vi "Run.vi"(8 "error in (no error)":errorcluster, 11 "Channel in":refnum<class "Channel.lvclass">) -> (0 "error out":errorcluster, 3 "Channel out":refnum<class "Channel.lvclass">)   [LabVIEW 2018, in "Channel.lvclass"]
doc: "Run the channel"
uses:
  Channel.lvclass
  Channel.lvclass/Channel.ctl
  Sim_Ixon_Ultra/Sim_Ixon_Ultra.lvclass
  C:/Users/Denis/Desktop/S4ACS/S4ACS/Simulated_CCD_Camera/Simulated Camera.lvclass
  State Machine/State Machine.lvclass
  Simulated_CCD_Camera/Simulated Camera.lvclass
  RxTx/RxTx.lvclass
  Server/Server.lvclass
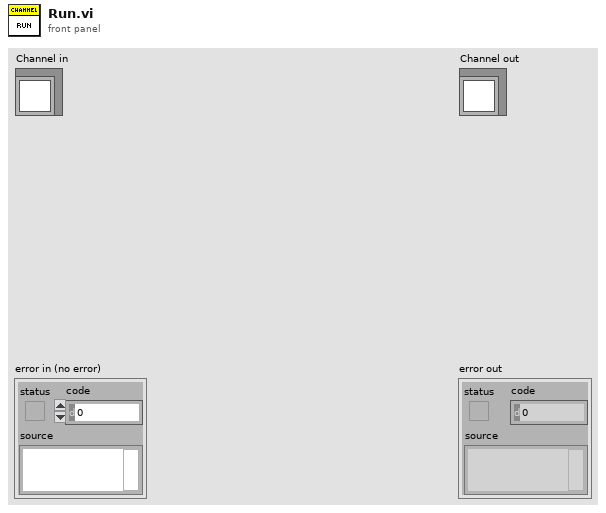
[diagram p1: front panel]
types:
  T1 = cluster{"PREAMP":u16, "READOUT_RATE":u16, "VERTICAL_SHIFT_SPEED":u16, "READ_MODE":u16, "VERTICAL_CLOCK_VOLTAGE":u16, "ACQUISITION_MODE":u16, "AD_CHANNEL":u16, "SHUTTER_TTL":u16, "SHUTTER_OPENING_TIME":u16, "SHUTTER_CLOSING_TIME":u16, "SHUTTER_MODE":u16, "TRIGGER_MODE":u16, "VBIN":u16, "INITIAL_LINE":u16, "INITIAL_COLUMN":u16, "FINAL_LINE":u16, "FINAL_COLUMN":u16, "HBIN":u16, "TEMP":u16, "COOLER_POWER_STATUS":u16}
  T2 = typedef "LVDateTimeRec.ctl" = cluster{"fractional second":dbl, "second":i32, "minute":i32, "hour":i32, "day of month":i32, "month":i32, "year":i32, "day of week":i32, "day of year":i32, "DST":i32}
  T3 = cluster{"Time Acq Started":u32, "Image delay":u64, "Last update - CCD config":timestamp, "SYSTEMTIME":T2, "Readout time":dbl, "Time acq finished":u32, "effective exptime":dbl}
  T4 = cluster{"FRAMES_DONE":u16, "CCD_STATUS":string, "CURRENT_TEMPERATURE":i16, "TEMPERATURE_STATUS":string, "FRAME_EXPOSURE_TIME":sgl, "SERIAL_NUMBER":u16, "ACQUIRING":bool, "POWER":bool}
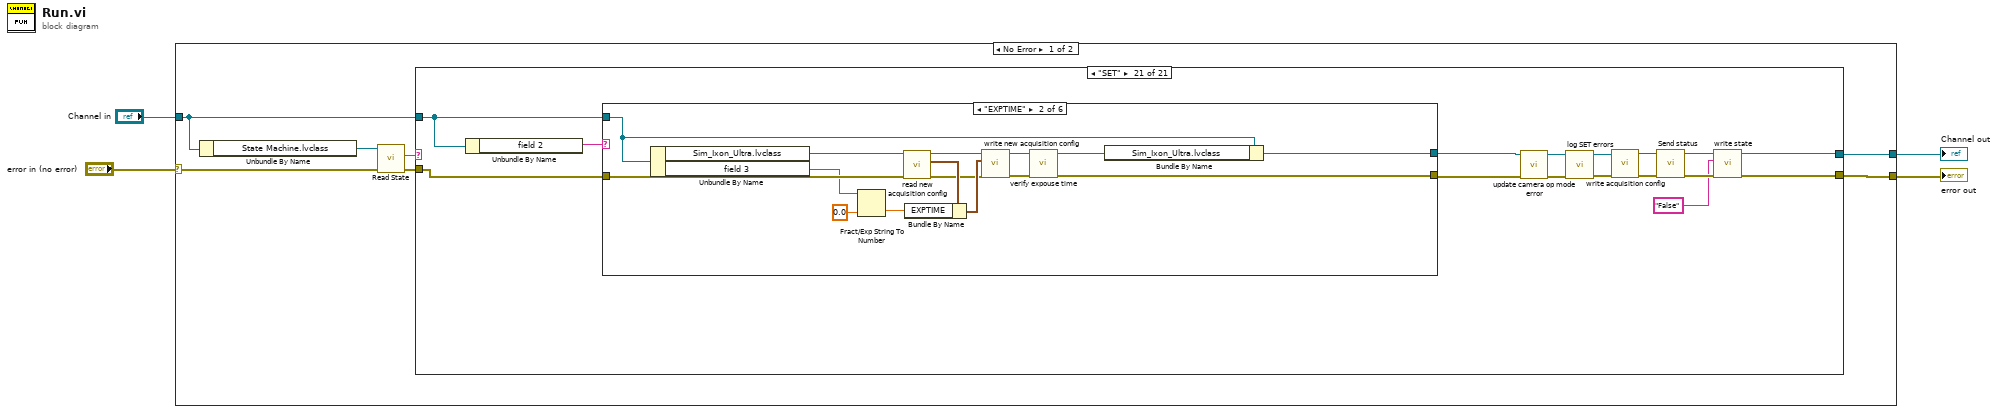
[diagram p0: block diagram]
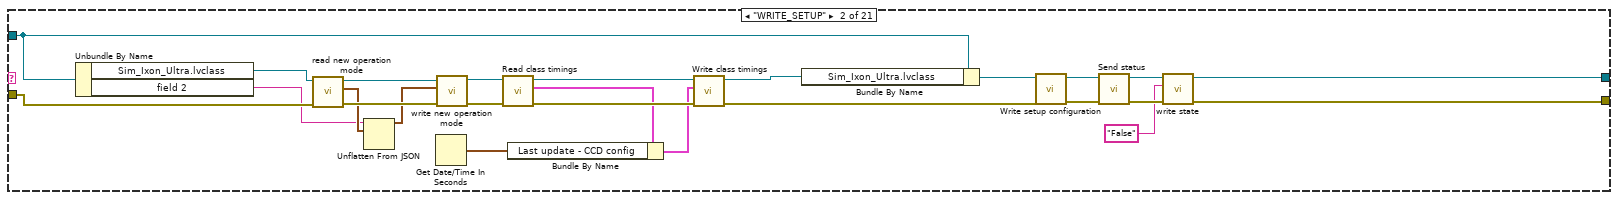
[diagram p3: hidden frame]
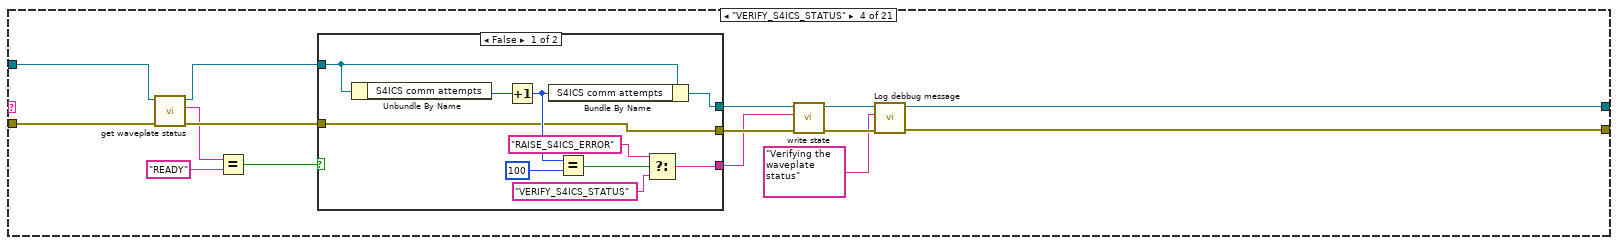
[diagram p5: hidden frame]
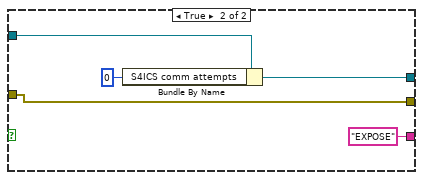
[diagram p6: hidden frame]
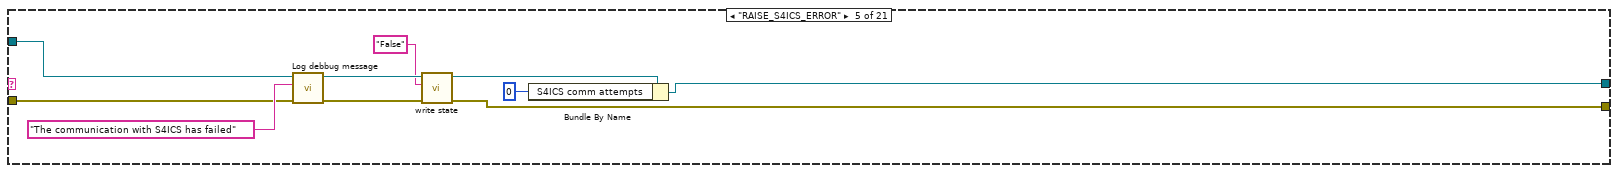
[diagram p7: hidden frame]
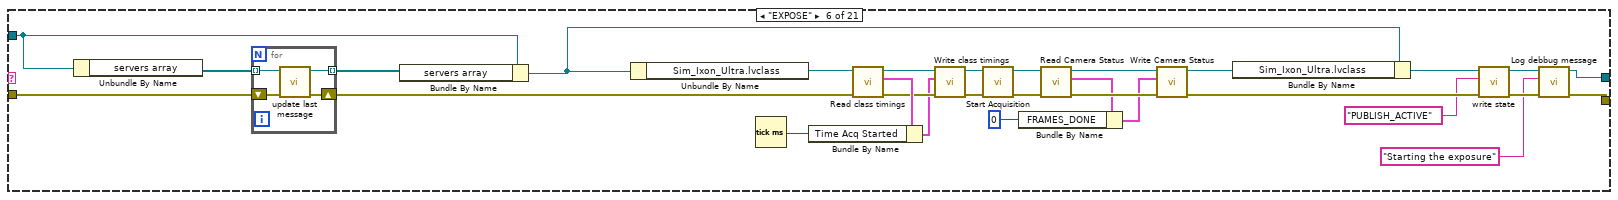
[diagram p8: hidden frame]
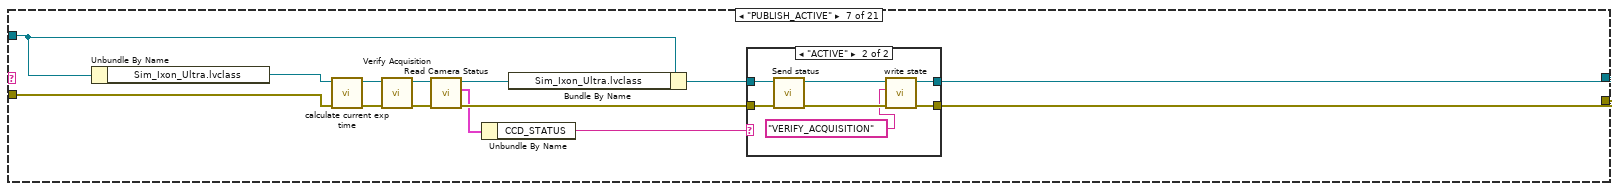
[diagram p9: hidden frame]
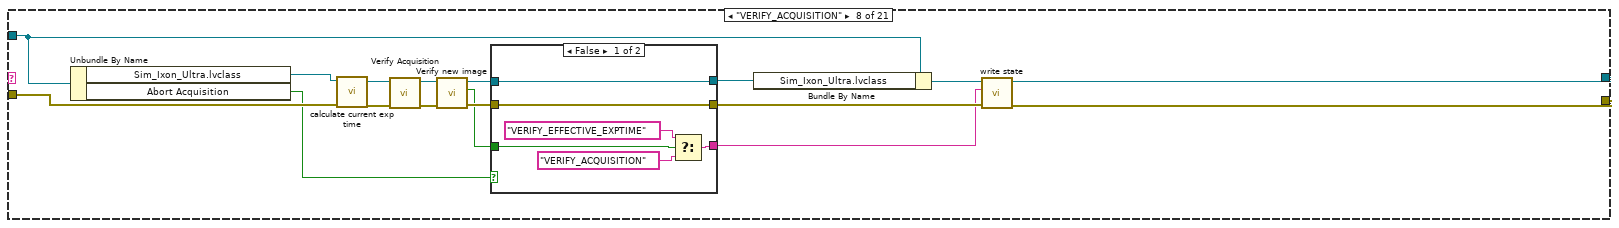
[diagram p11: hidden frame]
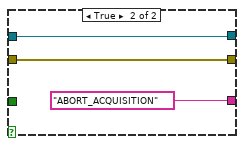
[diagram p12: hidden frame]
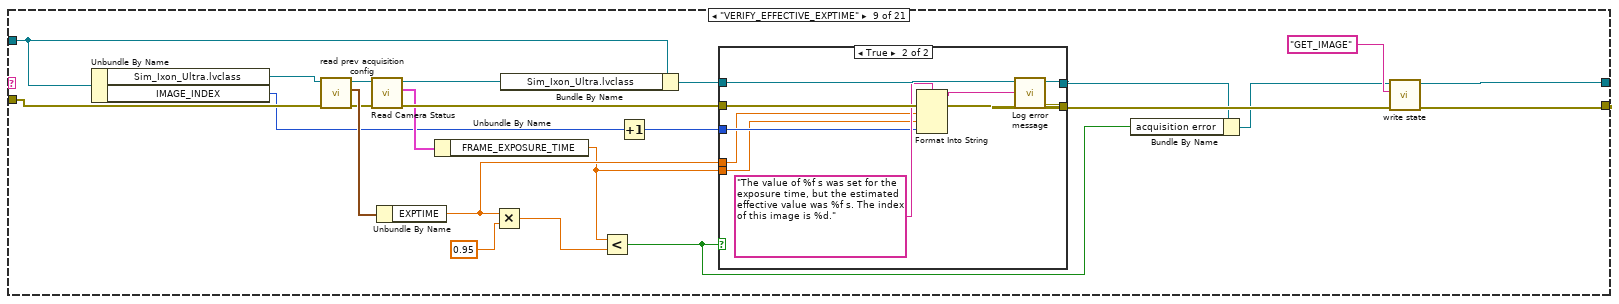
[diagram p13: hidden frame]
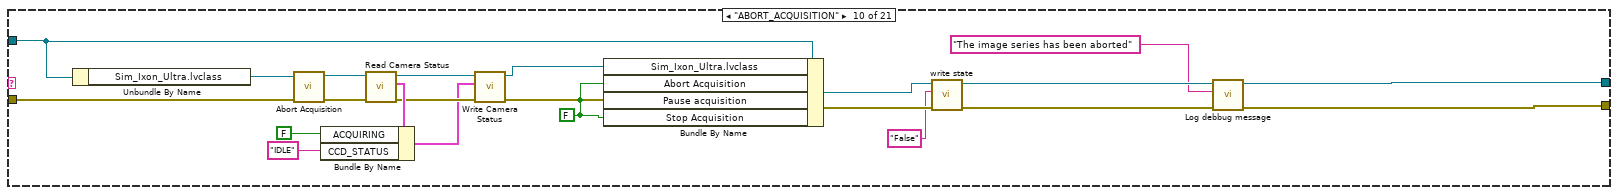
[diagram p15: hidden frame]
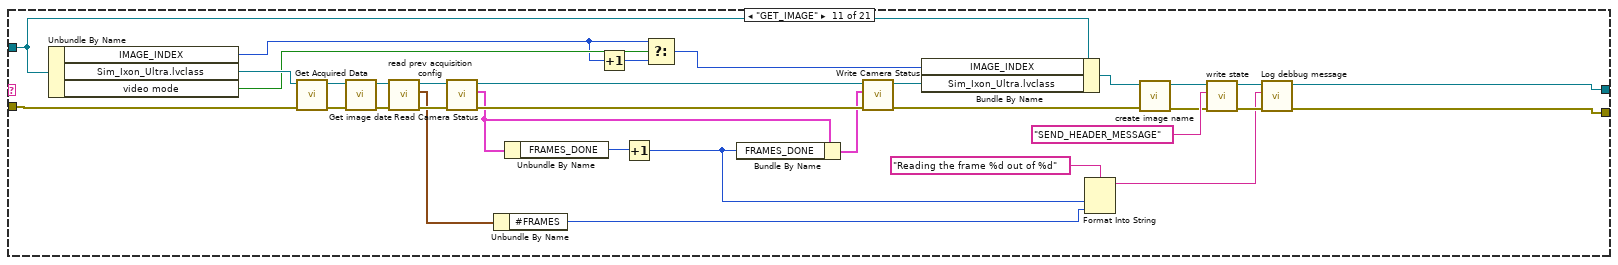
[diagram p16: hidden frame]
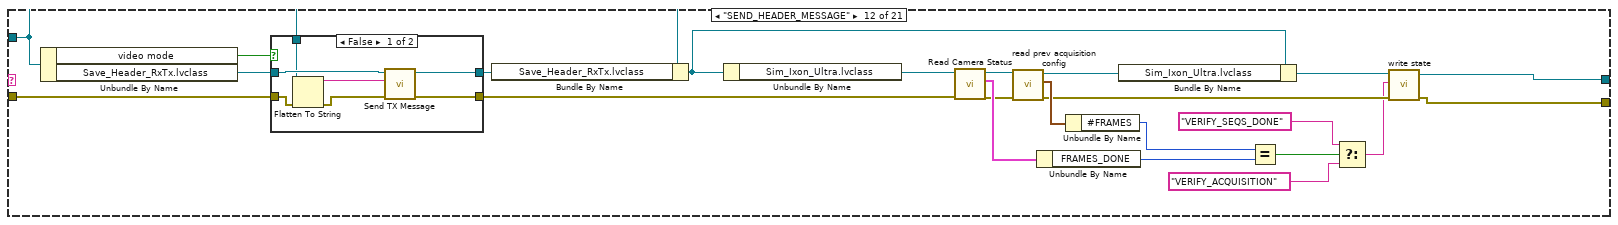
[diagram p17: hidden frame]
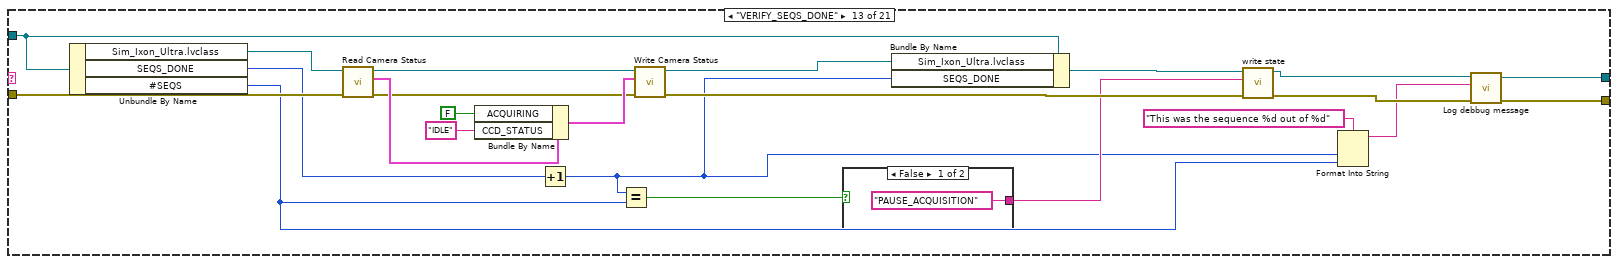
[diagram p19: hidden frame]
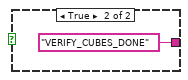
[diagram p20: hidden frame]
diagram:
  n1 = case shown="No Error" "error in (no error)" {
    selector: "error in (no error)" -> [w7 w466]
    tunnel: [w11 w466] -> w3
    tunnel: [w9 w465] -> w1
    tunnel: "Channel in" -> [w10 w465]
    frame No Error {
      n2 = Unbundle By Name(w10) -> ("State Machine.lvclass"=w8:refnum<class "State Machine.lvclass">)
      n3 = call-dynamic "Read State.vi"("error in (no error)"=w7, "State Machine in"=w8) -> ("error out"=w6:errorcluster, "State"=w5:string)  [unwired: 7 in, 1 out]
      n4 = case shown="\"SET\"" w5 {
        tunnel: w6 -> [w12 w37 w39 w43 w78 w97 w115 w141 w185 w210 w252 w262 w303 w324 w334 w339 w350 w378 w393 w399 w415]
        tunnel: [w12 w24 w39 w49 w72 w92 w125 w150 w183 w201 w235 w253 w292 w317 w330 w338 w346 w377 w395 w399 w411] -> w11
        tunnel: [w13 w25 w40 w50 w73 w93 w126 w151 w184 w202 w236 w254 w293 w316 w331 w337 w347 w376 w394 w400 w412] -> w9
        tunnel: w10 -> [w13 w38 w40 w45 w79 w104 w128 w154 w186 w209 w246 w255 w304 w325 w335 w340 w367 w379 w392 w400 w416]
        frame "False", Default {
        }
        frame "WRITE_SETUP" {
          n5 = Unbundle By Name(w38) -> ("Sim_Ixon_Ultra.lvclass"=w17:refnum<class "Sim_Ixon_Ultra.lvclass">, "field 2"=w26:string)
          n6 = call "read new operation mode.vi"("error in (no error)"=w37, "CCDCamera in"=w17) -> ("error out"=w35:errorcluster, "new operation mode"=w34:T1, "CCDCamera out"=w36:refnum<class "Sim_Ixon_Ultra.lvclass">)  [unwired: 7 in]
          n7 = Unflatten From JSON(JSON string=w26, type and defaults=w34) -> (value=w33:T1)  [unwired: 5 in, 1 out]
          n8 = Get Date/Time In Seconds() -> (seconds since 1Jan1904=w14:timestamp)
          n9 = call "write new operation mode.vi"("error in (no error)"=w35, "new operation mode"=w33, "CCDCamera in"=w36) -> ("error out"=w22:errorcluster, "CCDCamera out"=w23:refnum<class "Sim_Ixon_Ultra.lvclass">)  [unwired: 7 in]
          n10 = call "Read class timings.vi"("error in (no error)"=w22, "Simulated Camera in"=w23) -> ("error out"=w20:errorcluster, "class timings"=w16:T3, "Simulated Camera out"=w21:refnum<class "Sim_Ixon_Ultra.lvclass">)  [unwired: 7 in]
          n11 = Bundle By Name(cluster=w16, "Last update - CCD config"=w14) -> (w15:T3)
          n12 = call "Write class timings.vi"("error in (no error)"=w20, "class timings"=w15, "Simulated Camera in"=w21) -> ("error out"=w19:errorcluster, "Simulated Camera out"=w18:refnum<class "Sim_Ixon_Ultra.lvclass">)  [unwired: 7 in]
          n13 = Bundle By Name(cluster=w38, "Sim_Ixon_Ultra.lvclass"=w18) -> (w29:refnum<class "Channel.lvclass">)
          n14 = call "Write setup configuration.vi"("error in (no error)"=w19, "Channel in"=w29) -> ("error out"=w28:errorcluster, "Channel out"=w27:refnum<class "Channel.lvclass">)  [unwired: 8 in]
          n15 = call "Send status.vi"("error in (no error)"=w28, "Channel in"=w27) -> ("error out"=w31:errorcluster, "Channel out"=w32:refnum<class "Channel.lvclass">)  [unwired: 8 in]
          n16 = call "write state.vi"("error in (no error)"=w31, "state"="False", "Channel in"=w32) -> ("error out"=w24:errorcluster, "Channel out"=w25:refnum<class "Channel.lvclass">)  [unwired: 7 in]
        }
        frame "---------------------------------" {
        }
        frame "VERIFY_S4ICS_STATUS" {
          n17 = call "get waveplate status.vi"("error in (no error)"=w43, "Channel in"=w45) -> ("error out"=w42:errorcluster, "wp condition"=w41:string, "Channel out"=w44:refnum<class "Channel.lvclass">)  [unwired: 7 in]
          n18 = Equal?(x=w41, y="READY") -> (x = y?=w54:bool)
          n19 = case shown="False" w54 {
            tunnel: w44 -> [w65 w70]
            tunnel: w42 -> [w58 w69]
            tunnel: [w57 w68] -> w53
            tunnel: [w58 w69] -> w52
            tunnel: [w56 "EXPOSE" ("y")] -> w51
            frame False {
              n20 = Unbundle By Name(w65) -> ("S4ICS comm attempts"=w64:u8)
              n21 = Increment(x=w64) -> (x+1=w63:u8)
              n22 = Bundle By Name(cluster=w65, "S4ICS comm attempts"=w63) -> (w57:refnum<class "Channel.lvclass">)
              n23 = Equal?(x=w63, y=100) -> (x = y?=w61:bool)
              n24 = Select(t="RAISE_S4ICS_ERROR" ("y"), s=w61, f="VERIFY_S4ICS_STATUS" ("y")) -> (s? t:f=w56:string)
            }
            frame True {
              n25 = Bundle By Name(cluster=w70, "S4ICS comm attempts"=u8 0) -> (w68:refnum<class "Channel.lvclass">)
            }
          }
          n26 = call "write state.vi"("error in (no error)"=w52, "state"=w51, "Channel in"=w53) -> ("error out"=w48:errorcluster, "Channel out"=w47:refnum<class "Channel.lvclass">)  [unwired: 7 in]
          n27 = call "Log debbug message.vi"("error in (no error)"=w48, "String"="Verifying the waveplate status" ("y"), "Channel in"=w47) -> ("error out"=w49:errorcluster, "Channel out"=w50:refnum<class "Channel.lvclass">)  [unwired: 7 in]
        }
        frame "RAISE_S4ICS_ERROR" {
          n28 = call "Log debbug message.vi"("error in (no error)"=w78, "String"="The communication with S4ICS has failed", "Channel in"=w79) -> ("error out"=w75:errorcluster, "Channel out"=w76:refnum<class "Channel.lvclass">)  [unwired: 7 in]
          n29 = call "write state.vi"("error in (no error)"=w75, "state"="False", "Channel in"=w76) -> ("error out"=w72:errorcluster, "Channel out"=w74:refnum<class "Channel.lvclass">)  [unwired: 7 in]
          n30 = Bundle By Name(cluster=w74, "S4ICS comm attempts"=u8 0) -> (w73:refnum<class "Channel.lvclass">)
        }
        frame "EXPOSE" {
          n31 = Unbundle By Name(w104) -> ("servers array"=w95:refnum<class "Server.lvclass">[])
          n32 = for {
            tunnel: w95 -> [w111] mode=indexing
            shift-right: [w114] -> w88
            shift-left: w97 -> [w112]
            tunnel: [w113] -> w96 mode=indexing
            n33 = call "update last message.vi"("error in (no error)"=w112, "Server in"=w111) -> ("error out"=w114:errorcluster, "Server out"=w113:refnum<class "Server.lvclass">)  [unwired: 8 in]
          }
          n34 = Bundle By Name(cluster=w104, "servers array"=w96) -> (w103:refnum<class "Channel.lvclass">)
          n35 = Unbundle By Name(w103) -> ("Sim_Ixon_Ultra.lvclass"=w89:refnum<class "Sim_Ixon_Ultra.lvclass">)
          n36 = Tick Count (ms)() -> (millisecond timer value=w81:u32)
          n37 = call "Read class timings.vi"("error in (no error)"=w88, "Simulated Camera in"=w89) -> ("error out"=w84:errorcluster, "class timings"=w85:T3, "Simulated Camera out"=w83:refnum<class "Sim_Ixon_Ultra.lvclass">)  [unwired: 7 in]
          n38 = Bundle By Name(cluster=w85, "Time Acq Started"=w81) -> (w82:T3)
          n39 = call "Write class timings.vi"("error in (no error)"=w84, "class timings"=w82, "Simulated Camera in"=w83) -> ("error out"=w87:errorcluster, "Simulated Camera out"=w86:refnum<class "Sim_Ixon_Ultra.lvclass">)  [unwired: 7 in]
          n40 = call-dynamic "Start Acquisition.vi"("error in (no error)"=w87, "CCDCamera in"=w86) -> ("error out"=w98:errorcluster, "CCDCamera out"=w99:refnum<class "Sim_Ixon_Ultra.lvclass">)  [unwired: 8 in]
          n41 = call "Read Camera Status.vi"("error in (no error)"=w98, "CCDCamera in"=w99) -> ("error out"=w109:errorcluster, "camera status"=w107:T4, "CCDCamera out"=w108:refnum<class "Sim_Ixon_Ultra.lvclass">)  [unwired: 7 in]
          n42 = Bundle By Name(cluster=w107, "FRAMES_DONE"=u16 0) -> (w106:T4)
          n43 = call "Write Camera Status.vi"("error in (no error)"=w109, "camera status"=w106, "CCDCamera in"=w108) -> ("error out"=w101:errorcluster, "CCDCamera out"=w110:refnum<class "Sim_Ixon_Ultra.lvclass">)  [unwired: 7 in]
          n44 = Bundle By Name(cluster=w103, "Sim_Ixon_Ultra.lvclass"=w110) -> (w102:refnum<class "Channel.lvclass">)
          n45 = call "write state.vi"("error in (no error)"=w101, "state"="PUBLISH_ACTIVE", "Channel in"=w102) -> ("error out"=w91:errorcluster, "Channel out"=w94:refnum<class "Channel.lvclass">)  [unwired: 7 in]
          n46 = call "Log debbug message.vi"("error in (no error)"=w91, "String"="Starting the exposure", "Channel in"=w94) -> ("error out"=w92:errorcluster, "Channel out"=w93:refnum<class "Channel.lvclass">)  [unwired: 7 in]
        }
        frame "PUBLISH_ACTIVE" {
          n47 = Unbundle By Name(w128) -> ("Sim_Ixon_Ultra.lvclass"=w118:refnum<class "Sim_Ixon_Ultra.lvclass">)
          n48 = call-dynamic "calculate current exp time.vi"("error in (no error)"=w115, "CCDCamera in"=w118) -> ("error out"=w116:errorcluster, "CCDCamera out"=w117:refnum<class "Sim_Ixon_Ultra.lvclass">)  [unwired: 8 in]
          n49 = call-dynamic "Verify Acquisition.vi"("error in (no error)"=w116, "CCDCamera in"=w117) -> ("error out"=w119:errorcluster, "CCDCamera out"=w120:refnum<class "Sim_Ixon_Ultra.lvclass">)  [unwired: 8 in]
          n50 = call "Read Camera Status.vi"("error in (no error)"=w119, "CCDCamera in"=w120) -> ("error out"=w123:errorcluster, "camera status"=w122:T4, "CCDCamera out"=w124:refnum<class "Sim_Ixon_Ultra.lvclass">)  [unwired: 7 in]
          n51 = Unbundle By Name(w122) -> ("CCD_STATUS"=w121:string)
          n52 = Bundle By Name(cluster=w128, "Sim_Ixon_Ultra.lvclass"=w124) -> (w127:refnum<class "Channel.lvclass">)
          n53 = case shown="\"ACTIVE\"" w121 {
            tunnel: w127 -> [w130 w133]
            tunnel: [w130 w137] -> w126
            tunnel: [w129 w136] -> w125
            tunnel: w123 -> [w129 w132]
            frame "False", Default {
            }
            frame "ACTIVE" {
              n54 = call "Send status.vi"("error in (no error)"=w132, "Channel in"=w133) -> ("error out"=w135:errorcluster, "Channel out"=w134:refnum<class "Channel.lvclass">)  [unwired: 8 in]
              n55 = call "write state.vi"("error in (no error)"=w135, "state"="VERIFY_ACQUISITION", "Channel in"=w134) -> ("error out"=w136:errorcluster, "Channel out"=w137:refnum<class "Channel.lvclass">)  [unwired: 7 in]
            }
          }
        }
        frame "VERIFY_ACQUISITION" {
          n56 = Unbundle By Name(w154) -> ("Sim_Ixon_Ultra.lvclass"=w142:refnum<class "Sim_Ixon_Ultra.lvclass">, "Abort Acquisition"=w140:bool)
          n57 = call-dynamic "calculate current exp time.vi"("error in (no error)"=w141, "CCDCamera in"=w142) -> ("error out"=w143:errorcluster, "CCDCamera out"=w144:refnum<class "Sim_Ixon_Ultra.lvclass">)  [unwired: 8 in]
          n58 = call-dynamic "Verify Acquisition.vi"("error in (no error)"=w143, "CCDCamera in"=w144) -> ("error out"=w153:errorcluster, "CCDCamera out"=w152:refnum<class "Sim_Ixon_Ultra.lvclass">)  [unwired: 8 in]
          n59 = call-dynamic "Verify new image.vi"("error in (no error)"=w153, "CCDCamera in"=w152) -> ("error out"=w148:errorcluster, "New Images ?"=w138:bool, "CCDCamera out"=w149:refnum<class "Sim_Ixon_Ultra.lvclass">)  [unwired: 7 in]
          n60 = case shown="False" w140 {
            tunnel: w149 -> [w160 w163]
            tunnel: w148 -> [w159 w162]
            tunnel: [w160 w163] -> w147
            tunnel: [w159 w162] -> w145
            tunnel: [w156 "ABORT_ACQUISITION"] -> w139
            tunnel: w138 -> [w155 _]
            frame False {
              n61 = Select(t="VERIFY_EFFECTIVE_EXPTIME", s=w155, f="VERIFY_ACQUISITION") -> (s? t:f=w156:string)
            }
            frame True {
            }
          }
          n62 = Bundle By Name(cluster=w154, "Sim_Ixon_Ultra.lvclass"=w147) -> (w146:refnum<class "Channel.lvclass">)
          n63 = call "write state.vi"("error in (no error)"=w145, "state"=w139, "Channel in"=w146) -> ("error out"=w150:errorcluster, "Channel out"=w151:refnum<class "Channel.lvclass">)  [unwired: 7 in]
        }
        frame "VERIFY_EFFECTIVE_EXPTIME" {
          n64 = Unbundle By Name(w186) -> ("Sim_Ixon_Ultra.lvclass"=w165:refnum<class "Sim_Ixon_Ultra.lvclass">, "IMAGE_INDEX"=w164:u32)
          n65 = call "read prev acquisition config.vi"("error in (no error)"=w185, "Simulated_CCD_Camera in"=w165) -> ("error out"=w174:errorcluster, "Prev SET parameters"=w177:cluster{"EXPTIME":dbl, "#FRAMES":u32}, "Simulated_CCD_Camera out"=w176:refnum<class "Sim_Ixon_Ultra.lvclass">)  [unwired: 7 in]
          n66 = call "Read Camera Status.vi"("error in (no error)"=w174, "CCDCamera in"=w176) -> ("error out"=w173:errorcluster, "camera status"=w172:T4, "CCDCamera out"=w175:refnum<class "Sim_Ixon_Ultra.lvclass">)  [unwired: 7 in]
          n67 = Unbundle By Name(w177) -> ("EXPTIME"=w170:dbl)
          n68 = Unbundle By Name(w172) -> ("FRAME_EXPOSURE_TIME"=w169:sgl)
          n69 = Multiply(x=w170, y=0.95) -> (x*y=w178:dbl)
          n70 = Bundle By Name(cluster=w186, "Sim_Ixon_Ultra.lvclass"=w175) -> (w182:refnum<class "Channel.lvclass">)
          n71 = Less?(x=w169, y=w178) -> (x < y?=w166:bool)
          n72 = Increment(x=w164) -> (x+1=w171:u32)
          n73 = case shown="True" w166 {
            tunnel: w182 -> [w188 w198]
            tunnel: [w188 w197] -> w168
            tunnel: [w187 w196] -> w181
            tunnel: w173 -> [w187 w195]
            tunnel: w171 -> [_ w191]
            tunnel: w170 -> [_ w190]
            tunnel: w169 -> [_ w189]
            frame False {
            }
            frame True {
              n74 = Format Into String(format string="The value of %f s was set for the exposure time, but the estimated effective value was %f s. The index of this image is %d.", error in=w195, w190, w189, w191) -> (resulting string=w192:string, error out=w194:errorcluster)  [unwired: 1 in]
              n75 = call "Log error message.vi"("error in (no error)"=w194, "String"=w192, "Channel in"=w198) -> ("error out"=w196:errorcluster, "Channel out"=w197:refnum<class "Channel.lvclass">)  [unwired: 7 in]
            }
          }
          n76 = Bundle By Name(cluster=w168, "acquisition error"=w166) -> (w167:refnum<class "Channel.lvclass">)
          n77 = call "write state.vi"("error in (no error)"=w181, "state"="GET_IMAGE", "Channel in"=w167) -> ("error out"=w183:errorcluster, "Channel out"=w184:refnum<class "Channel.lvclass">)  [unwired: 7 in]
        }
        frame "ABORT_ACQUISITION" {
          w204 = FALSE ("Acquiring")
          n78 = Unbundle By Name(w209) -> ("Sim_Ixon_Ultra.lvclass"=w211:refnum<class "Sim_Ixon_Ultra.lvclass">)
          n79 = call-dynamic "Abort Acquisition.vi"("error in (no error)"=w210, "CCDCamera in"=w211) -> ("error out"=w216:errorcluster, "CCDCamera out"=w217:refnum<class "Sim_Ixon_Ultra.lvclass">)  [unwired: 8 in]
          n80 = call "Read Camera Status.vi"("error in (no error)"=w216, "CCDCamera in"=w217) -> ("error out"=w214:errorcluster, "camera status"=w219:T4, "CCDCamera out"=w215:refnum<class "Sim_Ixon_Ultra.lvclass">)  [unwired: 7 in]
          n81 = Bundle By Name(cluster=w219, "ACQUIRING"=FALSE ("Acquiring"), "CCD_STATUS"="IDLE" ("STATUS")) -> (w213:T4)
          n82 = call "Write Camera Status.vi"("error in (no error)"=w214, "camera status"=w213, "CCDCamera in"=w215) -> ("error out"=w206:errorcluster, "CCDCamera out"=w208:refnum<class "Sim_Ixon_Ultra.lvclass">)  [unwired: 7 in]
          n83 = Bundle By Name(cluster=w209, "Sim_Ixon_Ultra.lvclass"=w208, "Abort Acquisition"=w204, "Pause acquisition"=w204, "Stop Acquisition"=w204) -> (w207:refnum<class "Channel.lvclass">)
          n84 = call "write state.vi"("error in (no error)"=w206, "state"="False", "Channel in"=w207) -> ("error out"=w200:errorcluster, "Channel out"=w203:refnum<class "Channel.lvclass">)  [unwired: 7 in]
          n85 = call "Log debbug message.vi"("error in (no error)"=w200, "String"="The image series has been aborted", "Channel in"=w203) -> ("error out"=w201:errorcluster, "Channel out"=w202:refnum<class "Channel.lvclass">)  [unwired: 7 in]
        }
        frame "GET_IMAGE" {
          n86 = Unbundle By Name(w246) -> ("IMAGE_INDEX"=w221:u32, "Sim_Ixon_Ultra.lvclass"=w241:refnum<class "Sim_Ixon_Ultra.lvclass">, "video mode"=w239:bool)
          n87 = call-dynamic "Get Acquired Data.vi"("error in (no error)"=w252, "CCDCamera in"=w241) -> ("error out"=w242:errorcluster, "CCDCamera out"=w243:refnum<class "Sim_Ixon_Ultra.lvclass">)  [unwired: 8 in]
          n88 = call-dynamic "Get image date.vi"("error in (no error)"=w242, "Simulated_CCD_Camera in"=w243) -> ("error out"=w230:errorcluster, "Simulated_CCD_Camera out"=w227:refnum<class "Sim_Ixon_Ultra.lvclass">)  [unwired: 8 in]
          n89 = call "read prev acquisition config.vi"("error in (no error)"=w230, "Simulated_CCD_Camera in"=w227) -> ("error out"=w229:errorcluster, "Prev SET parameters"=w226:cluster{"EXPTIME":dbl, "#FRAMES":u32}, "Simulated_CCD_Camera out"=w228:refnum<class "Sim_Ixon_Ultra.lvclass">)  [unwired: 7 in]
          n90 = call "Read Camera Status.vi"("error in (no error)"=w229, "CCDCamera in"=w228) -> ("error out"=w251:errorcluster, "camera status"=w247:T4, "CCDCamera out"=w250:refnum<class "Sim_Ixon_Ultra.lvclass">)  [unwired: 7 in]
          n91 = Unbundle By Name(w226) -> ("#FRAMES"=w225:u32)
          n92 = Unbundle By Name(w247) -> ("FRAMES_DONE"=w249:u16)
          n93 = Increment(x=w221) -> (x+1=w240:u32)
          n94 = Increment(x=w249) -> (x+1=w231:u16)
          n95 = Select(t=w221, s=w239, f=w240) -> (s? t:f=w220:u32)
          n96 = Bundle By Name(cluster=w247, "FRAMES_DONE"=w231) -> (w248:T4)
          n97 = call "Write Camera Status.vi"("error in (no error)"=w251, "camera status"=w248, "CCDCamera in"=w250) -> ("error out"=w244:errorcluster, "CCDCamera out"=w245:refnum<class "Sim_Ixon_Ultra.lvclass">)  [unwired: 7 in]
          n98 = Bundle By Name(cluster=w246, "IMAGE_INDEX"=w220, "Sim_Ixon_Ultra.lvclass"=w245) -> (w224:refnum<class "Channel.lvclass">)
          n99 = Format Into String(format string="Reading the frame %d out of %d", w231, w225) -> (resulting string=w232:string)  [unwired: 2 in, 1 out]
          n100 = call "create image name.vi"("error in (no error)"=w244, "Channel in"=w224) -> ("error out"=w222:errorcluster, "Channel out"=w223:refnum<class "Channel.lvclass">)  [unwired: 8 in]
          n101 = call "write state.vi"("error in (no error)"=w222, "state"="SEND_HEADER_MESSAGE", "Channel in"=w223) -> ("error out"=w234:errorcluster, "Channel out"=w237:refnum<class "Channel.lvclass">)  [unwired: 7 in]
          n102 = call "Log debbug message.vi"("error in (no error)"=w234, "String"=w232, "Channel in"=w237) -> ("error out"=w235:errorcluster, "Channel out"=w236:refnum<class "Channel.lvclass">)  [unwired: 7 in]
        }
        frame "SEND_HEADER_MESSAGE" {
          n103 = Unbundle By Name(w255) -> ("video mode"=w259:bool, "Save_Header_RxTx.lvclass"=w263:refnum<class "RxTx.lvclass">)
          n104 = case shown="False" w259 {
            tunnel: w263 -> [w282 w284]
            tunnel: w262 -> [w281 w283]
            tunnel: [w277 w284] -> w261
            tunnel: [w276 w283] -> w260
            tunnel: w255 -> [w280 _]
            frame False {
              n105 = Flatten To String(anything=w280, error in (no error)=w281) -> (data string=w278:string, error out=w279:errorcluster)  [unwired: 2 in, 1 out]
              n106 = call "Send TX Message.vi"("error in (no error)"=w279, "message"=w278, "RxTx in"=w282) -> ("error out"=w276:errorcluster, "RxTx out"=w277:refnum<class "RxTx.lvclass">)  [unwired: 7 in]
            }
            frame True {
            }
          }
          n107 = Bundle By Name(cluster=w255, "Save_Header_RxTx.lvclass"=w261) -> (w273:refnum<class "Channel.lvclass">)
          n108 = Unbundle By Name(w273) -> ("Sim_Ixon_Ultra.lvclass"=w270:refnum<class "Sim_Ixon_Ultra.lvclass">)
          n109 = call "Read Camera Status.vi"("error in (no error)"=w260, "CCDCamera in"=w270) -> ("error out"=w266:errorcluster, "camera status"=w269:T4, "CCDCamera out"=w268:refnum<class "Sim_Ixon_Ultra.lvclass">)  [unwired: 7 in]
          n110 = call "read prev acquisition config.vi"("error in (no error)"=w266, "Simulated_CCD_Camera in"=w268) -> ("error out"=w257:errorcluster, "Prev SET parameters"=w265:cluster{"EXPTIME":dbl, "#FRAMES":u32}, "Simulated_CCD_Camera out"=w267:refnum<class "Sim_Ixon_Ultra.lvclass">)  [unwired: 7 in]
          n111 = Unbundle By Name(w269) -> ("FRAMES_DONE"=w275:u16)
          n112 = Unbundle By Name(w265) -> ("#FRAMES"=w264:u32)
          n113 = Bundle By Name(cluster=w273, "Sim_Ixon_Ultra.lvclass"=w267) -> (w258:refnum<class "Channel.lvclass">)
          n114 = Equal?(x=w264, y=w275) -> (x = y?=w274:bool)
          n115 = Select(t="VERIFY_SEQS_DONE", s=w274, f="VERIFY_ACQUISITION") -> (s? t:f=w256:string)
          n116 = call "write state.vi"("error in (no error)"=w257, "state"=w256, "Channel in"=w258) -> ("error out"=w253:errorcluster, "Channel out"=w254:refnum<class "Channel.lvclass">)  [unwired: 7 in]
        }
        frame "VERIFY_SEQS_DONE" {
          n117 = Unbundle By Name(w304) -> ("Sim_Ixon_Ultra.lvclass"=w288:refnum<class "Sim_Ixon_Ultra.lvclass">, "SEQS_DONE"=w286:u16, "#SEQS"=w287:u32)
          n118 = call "Read Camera Status.vi"("error in (no error)"=w303, "CCDCamera in"=w288) -> ("error out"=w300:errorcluster, "camera status"=w307:T4, "CCDCamera out"=w301:refnum<class "Sim_Ixon_Ultra.lvclass">)  [unwired: 7 in]
          n119 = Bundle By Name(cluster=w307, "ACQUIRING"=FALSE, "CCD_STATUS"="IDLE") -> (w306:T4)
          n120 = Increment(x=w286) -> (x+1=w285:u16)
          n121 = Equal?(x=w285, y=w287) -> (x = y?=w305:bool)
          n122 = call "Write Camera Status.vi"("error in (no error)"=w300, "camera status"=w306, "CCDCamera in"=w301) -> ("error out"=w296:errorcluster, "CCDCamera out"=w302:refnum<class "Sim_Ixon_Ultra.lvclass">)  [unwired: 7 in]
          n123 = case shown="False" w305 {
            tunnel: ["PAUSE_ACQUISITION" "VERIFY_CUBES_DONE"] -> w295
            frame False {
            }
            frame True {
            }
          }
          n124 = Bundle By Name(cluster=w304, "Sim_Ixon_Ultra.lvclass"=w302, "SEQS_DONE"=w285) -> (w297:refnum<class "Channel.lvclass">)
          n125 = call "write state.vi"("error in (no error)"=w296, "state"=w295, "Channel in"=w297) -> ("error out"=w291:errorcluster, "Channel out"=w294:refnum<class "Channel.lvclass">)  [unwired: 7 in]
          n126 = Format Into String(format string="This was the sequence %d out of %d", w285, w287) -> (resulting string=w289:string)  [unwired: 2 in, 1 out]
          n127 = call "Log debbug message.vi"("error in (no error)"=w291, "String"=w289, "Channel in"=w294) -> ("error out"=w292:errorcluster, "Channel out"=w293:refnum<class "Channel.lvclass">)  [unwired: 7 in]
        }
        frame "VERIFY_CUBES_DONE" {
          n128 = Unbundle By Name(w325) -> ("CYCLES_DONE"=w311:u16, "#CYCLES"=w312:u32)
          n129 = Increment(x=w311) -> (x+1=w310:u16)
          n130 = Equal?(x=w310, y=w312) -> (x = y?=w323:bool)
          n131 = case shown="True" w323 {
            tunnel: ["PAUSE_ACQUISITION" "LOG_END_OF_SERIES"] -> w319
            frame False {
            }
            frame True {
            }
          }
          n132 = Bundle By Name(cluster=w325, "CYCLES_DONE"=w310) -> (w322:refnum<class "Channel.lvclass">)
          n133 = call "write state.vi"("error in (no error)"=w324, "state"=w319, "Channel in"=w322) -> ("error out"=w320:errorcluster, "Channel out"=w321:refnum<class "Channel.lvclass">)  [unwired: 7 in]
          n134 = Format Into String(format string="This was the cycle %d out of %d", w310, w312) -> (resulting string=w314:string)  [unwired: 2 in, 1 out]
          n135 = call "Send status.vi"("error in (no error)"=w320, "Channel in"=w321) -> ("error out"=w318:errorcluster, "Channel out"=w315:refnum<class "Channel.lvclass">)  [unwired: 8 in]
          n136 = call "Log debbug message.vi"("error in (no error)"=w318, "String"=w314, "Channel in"=w315) -> ("error out"=w317:errorcluster, "Channel out"=w316:refnum<class "Channel.lvclass">)  [unwired: 7 in]
        }
        frame "LOG_END_OF_SERIES" {
          n137 = call "write state.vi"("error in (no error)"=w334, "state"="False", "Channel in"=w335) -> ("error out"=w332:errorcluster, "Channel out"=w333:refnum<class "Channel.lvclass">)  [unwired: 7 in]
          n138 = call "Log info message.vi"("error in (no error)"=w332, "String"="The acquisition of the image series has been finished", "Channel in"=w333) -> ("error out"=w330:errorcluster, "Channel out"=w331:refnum<class "Channel.lvclass">)  [unwired: 7 in]
        }
        frame "PAUSE_ACQUISITION" {
          n139 = Unbundle By Name(w340) -> ("Pause acquisition"=w343:bool)
          n140 = Select(t="PAUSE_ACQUISITION", s=w343, f="STOP_ACQUISITION") -> (s? t:f=w336:string)
          n141 = call "write state.vi"("error in (no error)"=w339, "state"=w336, "Channel in"=w340) -> ("error out"=w338:errorcluster, "Channel out"=w337:refnum<class "Channel.lvclass">)  [unwired: 7 in]
        }
        frame "STOP_ACQUISITION" {
          n142 = Unbundle By Name(w367) -> ("Stop Acquisition"=w344:bool)
          n143 = Bundle By Name(cluster=w367, "Stop Acquisition"=FALSE) -> (w353:refnum<class "Channel.lvclass">)
          n144 = Select(t="False", s=w344, f="WAIT_EXPOSE_COMMAND") -> (s? t:f=w349:string)
          n145 = call "write state.vi"("error in (no error)"=w350, "state"=w349, "Channel in"=w353) -> ("error out"=w351:errorcluster, "Channel out"=w352:refnum<class "Channel.lvclass">)  [unwired: 7 in]
          n146 = Unbundle By Name(w352) -> ("Sim_Ixon_Ultra.lvclass"=w363:refnum<class "Sim_Ixon_Ultra.lvclass">)
          n147 = Not(x=w344) -> (.not. x?=w354:bool)
          n148 = Select(t="WAITING_EXPOSE_COMMAND" ("CCD_STATUS"), s=w354, f="IDLE" ("CCD_STATUS")) -> (s? t:f=w357:string)
          n149 = call "Read Camera Status.vi"("error in (no error)"=w351, "CCDCamera in"=w363) -> ("error out"=w360:errorcluster, "camera status"=w362:T4, "CCDCamera out"=w359:refnum<class "Sim_Ixon_Ultra.lvclass">)  [unwired: 7 in]
          n150 = Bundle By Name(cluster=w362, "CCD_STATUS"=w357) -> (w361:T4)
          n151 = call "Write Camera Status.vi"("error in (no error)"=w360, "camera status"=w361, "CCDCamera in"=w359) -> ("error out"=w345:errorcluster, "CCDCamera out"=w358:refnum<class "Sim_Ixon_Ultra.lvclass">)  [unwired: 7 in]
          n152 = Bundle By Name(cluster=w352, "Sim_Ixon_Ultra.lvclass"=w358) -> (w348:refnum<class "Channel.lvclass">)
          n153 = case shown="True" w344 {
            tunnel: w348 -> [w369 w374]
            tunnel: [w369 w373] -> w347
            tunnel: [w368 w372] -> w346
            tunnel: w345 -> [w368 w371]
            frame False {
            }
            frame True {
              n154 = call "Log debbug message.vi"("error in (no error)"=w371, "String"="The acquisition has been stopped", "Channel in"=w374) -> ("error out"=w372:errorcluster, "Channel out"=w373:refnum<class "Channel.lvclass">)  [unwired: 7 in]
            }
          }
        }
        frame "WAIT_EXPOSE_COMMAND" {
          n155 = Unbundle By Name(w379) -> ("wait expose command"=w380:bool)
          n156 = Select(t="STOP_ACQUISITION", s=w380, f="RESET_#SEQS") -> (s? t:f=w375:string)
          n157 = call "write state.vi"("error in (no error)"=w378, "state"=w375, "Channel in"=w379) -> ("error out"=w377:errorcluster, "Channel out"=w376:refnum<class "Channel.lvclass">)  [unwired: 7 in]
        }
        frame "RESET_#SEQS" {
          n158 = call "choose firs acquisition state.vi"("error in (no error)"=w393, "Channel in"=w392) -> ("error out"=w390:errorcluster, "verify S4ICS status"=w386:bool, "Channel out"=w391:refnum<class "Channel.lvclass">)  [unwired: 7 in]
          n159 = Select(t="VERIFY_S4ICS_STATUS", s=w386, f="EXPOSE") -> (s? t:f=w388:string)
          n160 = call "write state.vi"("error in (no error)"=w390, "state"=w388, "Channel in"=w391) -> ("error out"=w395:errorcluster, "Channel out"=w396:refnum<class "Channel.lvclass">)  [unwired: 7 in]
          n161 = Unbundle By Name(w396) -> ("#SEQS"=w385:u32, "SEQS_DONE"=w383:u16)
          n162 = Equal?(x=w383, y=w385) -> (x = y?=w398:bool)
          n163 = Select(t=0, s=w398, f=w383) -> (s? t:f=w384:i32)
          n164 = Bundle By Name(cluster=w396, "SEQS_DONE"=w384) -> (w394:refnum<class "Channel.lvclass">)
        }
        frame "------------------------------" {
        }
        frame "SET" {
          n165 = Unbundle By Name(w416) -> ("field 2"=w407:string)
          n166 = case shown="\"EXPTIME\"" w407 {
            tunnel: [w418 w420 w435 w451 w457 w464] -> w404
            tunnel: w416 -> [w418 w433 w448 w454 w459 w461]
            tunnel: [w417 w419 w434 w449 w455 w463] -> w401
            tunnel: w415 -> [w417 w429 w445 w449 w455 w463]
            frame "False", Default {
            }
            frame "EXPTIME" {
              n167 = Unbundle By Name(w433) -> ("Sim_Ixon_Ultra.lvclass"=w430:refnum<class "Sim_Ixon_Ultra.lvclass">, "field 3"=w421:string)
              n168 = Fract/Exp String To Number(string=w421, default (0 dbl)=0.0) -> (number=w431:dbl)  [unwired: 2 in, 1 out]
              n169 = call "read new acquisition config.vi"("error in (no error)"=w429, "Simulated_CCD_Camera in"=w430) -> ("error out"=w425:errorcluster, "New SET parameters"=w428:cluster{"EXPTIME":dbl, "#FRAMES":u32}, "Simulated_CCD_Camera out"=w426:refnum<class "Sim_Ixon_Ultra.lvclass">)  [unwired: 7 in]
              n170 = Bundle By Name(cluster=w428, "EXPTIME"=w431) -> (w427:cluster{"EXPTIME":dbl, "#FRAMES":u32})
              n171 = call "write new acquisition config.vi"("error in (no error)"=w425, "new acquisition configuration"=w427, "Simulated_CCD_Camera in"=w426) -> ("error out"=w424:errorcluster, "Simulated_CCD_Camera out"=w422:refnum<class "Sim_Ixon_Ultra.lvclass">)  [unwired: 7 in]
              n172 = call-dynamic "verify expouse time.vi"("error in (no error)"=w424, "Simulated_CCD_Camera in"=w422) -> ("error out"=w419:errorcluster, "Simulated_CCD_Camera out"=w423:refnum<class "Sim_Ixon_Ultra.lvclass">)  [unwired: 8 in]
              n173 = Bundle By Name(cluster=w433, "Sim_Ixon_Ultra.lvclass"=w423) -> (w420:refnum<class "Channel.lvclass">)
            }
            frame "#FRAMES" {
              n174 = Unbundle By Name(w448) -> ("Sim_Ixon_Ultra.lvclass"=w446:refnum<class "Sim_Ixon_Ultra.lvclass">, "field 3"=w436:string)
              n175 = Fract/Exp String To Number(string=w436, default (0 dbl)=u32 0) -> (number=w437:u32)  [unwired: 2 in, 1 out]
              n176 = call "read new acquisition config.vi"("error in (no error)"=w445, "Simulated_CCD_Camera in"=w446) -> ("error out"=w441:errorcluster, "New SET parameters"=w444:cluster{"EXPTIME":dbl, "#FRAMES":u32}, "Simulated_CCD_Camera out"=w442:refnum<class "Sim_Ixon_Ultra.lvclass">)  [unwired: 7 in]
              n177 = Bundle By Name(cluster=w444, "#FRAMES"=w437) -> (w443:cluster{"EXPTIME":dbl, "#FRAMES":u32})
              n178 = call "write new acquisition config.vi"("error in (no error)"=w441, "new acquisition configuration"=w443, "Simulated_CCD_Camera in"=w442) -> ("error out"=w439:errorcluster, "Simulated_CCD_Camera out"=w440:refnum<class "Sim_Ixon_Ultra.lvclass">)  [unwired: 7 in]
              n179 = call "verify #frames.vi"("error in (no error)"=w439, "Simulated_CCD_Camera in"=w440) -> ("error out"=w434:errorcluster, "Simulated_CCD_Camera out"=w438:refnum<class "Sim_Ixon_Ultra.lvclass">)  [unwired: 8 in]
              n180 = Bundle By Name(cluster=w448, "Sim_Ixon_Ultra.lvclass"=w438) -> (w435:refnum<class "Channel.lvclass">)
            }
            frame "#CYCLES" {
              n181 = Unbundle By Name(w454) -> ("field 3"=w452:string)
              n182 = Fract/Exp String To Number(string=w452, default (0 dbl)=u32 0) -> (number=w450:u32)  [unwired: 2 in, 1 out]
              n183 = Bundle By Name(cluster=w454, "#CYCLES"=w450) -> (w451:refnum<class "Channel.lvclass">)
            }
            frame "WAVEPLATE_POS" {
              n184 = Unbundle By Name(w459) -> ("field 3"=w458:string)
              n185 = Decimal String To Number(string=w458) -> (number=w456:i32)  [unwired: 2 in, 1 out]
              n186 = Bundle By Name(cluster=w459, "WAVEPLATE_POS"=w456) -> (w457:refnum<class "Channel.lvclass">)
            }
            frame "SUFFIX" {
              n187 = Unbundle By Name(w461) -> ("suffix"=w460:string)
              n188 = To Lower Case(string=w460) -> (all lower case string=w462:string)
              n189 = Bundle By Name(cluster=w461, "suffix"=w462) -> (w464:refnum<class "Channel.lvclass">)
            }
          }
          n190 = call "update camera op mode error.vi"("error in (no error)"=w401, "Channel in"=w404) -> ("error out"=w405:errorcluster, "Channel out"=w406:refnum<class "Channel.lvclass">)  [unwired: 8 in]
          n191 = call "log SET errors.vi"("error in (no error)"=w405, "Channel in"=w406) -> ("error out"=w402:errorcluster, "Channel out"=w403:refnum<class "Channel.lvclass">)  [unwired: 8 in]
          n192 = call "write acquisition config.vi"("error in (no error)"=w402, "Channel in"=w403) -> ("error out"=w409:errorcluster, "Channel out"=w408:refnum<class "Channel.lvclass">)  [unwired: 8 in]
          n193 = call "Send status.vi"("error in (no error)"=w409, "Channel in"=w408) -> ("error out"=w413:errorcluster, "Channel out"=w414:refnum<class "Channel.lvclass">)  [unwired: 8 in]
          n194 = call "write state.vi"("error in (no error)"=w413, "state"="False", "Channel in"=w414) -> ("error out"=w411:errorcluster, "Channel out"=w412:refnum<class "Channel.lvclass">)  [unwired: 7 in]
        }
      }
    }
    frame Error {
    }
  }
  "error out" <- w3
  "Channel out" <- w1
